vi "CheckBool.vi"(11 "Input Boolean":bool) -> (3 "Boolean Changed?":bool)   [LabVIEW 2013]
doc: "Checks to see if the boolean input has changed. If so, return true."
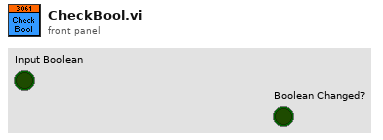
[diagram p1: front panel]
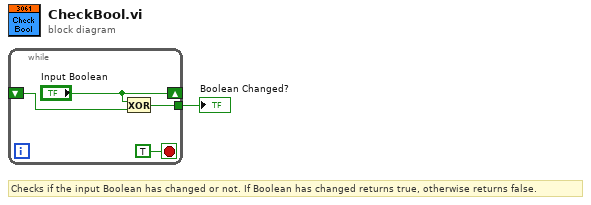
[diagram p0: block diagram]
diagram:
  # "Checks if the input Boolean has changed or not. If Boolean has changed returns true, otherwise returns false."
  n1 = while {
    tunnel: [w4] -> w1
    shift-right: ["Input Boolean"] -> _
    shift-left: _ -> [w2]
    stop <- TRUE stop-if-true
    n2 = Exclusive Or(1:w2, 2:"Input Boolean") -> (0:w4:bool)
  }
  "Boolean Changed?" <- w1
